vi "标准化行结束符.vi"(4 "End Of Line (Native)":T1(ring) caption="EOL(Native)", 7 "String In":string caption="字符串输入") -> (2 "String Out":string caption="字符串输出")   [LabVIEW 2012]
doc: "Converts the line endings of <B>String In</B> from whatever they are to the type indicated in <B>End Of Line</B>.\n\n<B>String In</B> - The string to convert.\n<B>String Out</B> - The string with the line endings changed.\n<B>End Of Line</B> - The type of line ending to convert to.\n\n<B>Native</B> is the native line ending (ie DOS \\r\\n, UNIX \\n, Mac \\r). <B>Native Command Line</B> is the appropriate of line ending when working with the command line."
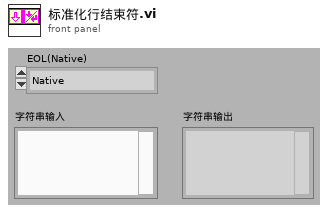
[diagram p1: front panel]
types:
  T1 = enum16{"Native", "Native Command Line", "UNIX", "Macintosh", "DOS"}
  T2 = enum32{"invalid OS target", "Mac OS", "Windows 3.1", "Windows 95/NT", "Solaris 1", "Solaris 2", "HP-UX", "PowerMAX", "Linux", "Irix", "Rhapsody", "BeOS", "AIX", "OSF1", "VxWorks", "PharLap", "Carbon"}
  T3 = enum32{"invalid OS target", "Mac OS", "Windows 3.1", "Windows 95/NT", "Solaris 1", "Solaris 2", "HP-UX", "PowerMAX", "Linux", "Irix", "Rhapsody", "BeOS", "AIX", "OSF1", "VxWorks", "PharLap", "Carbon", "RTX", "Windows x64", "Linux x64"}
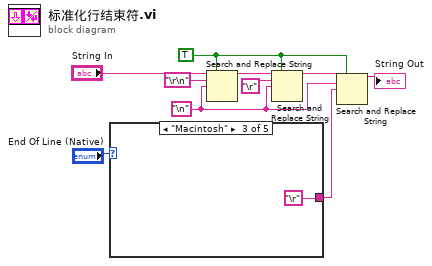
[diagram p0: block diagram]
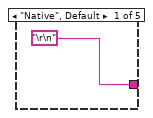
[diagram p2: hidden frame]
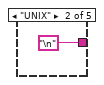
[diagram p3: hidden frame]
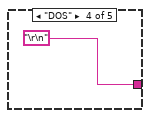
[diagram p4: hidden frame]
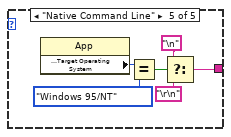
[diagram p5: hidden frame]
diagram:
  w3 = "\n" ("search string")
  w4 = TRUE ("replace all? (F)")
  n1 = case shown="\"Macintosh\"" "End Of Line (Native)" {
    tunnel: ["\r\n" "\n" "\r" "\r\n" w15] -> w2
    frame "Native", Default {
    }
    frame "UNIX" {
    }
    frame "Macintosh" {
    }
    frame "DOS" {
    }
    frame "Native Command Line" {
      n2 = property class="App"() -> ("Application:Target Operating System"=w20:T3)  [unwired: 2 in, 2 out]
      n3 = Equal?(x=w20, y=T2."Windows 95/NT" ("Application:Target Operating System")) -> (x = y?=w18:bool)
      n4 = Select(t="\n" ("search string"), s=w18, f="\r\n") -> (s? t:f=w15:string)
    }
  }
  n5 = Search and Replace String(replace all?=w4, input string="String In", search string="\r\n", replace string=w3) -> (result string=w8:string)  [unwired: 4 in, 3 out]
  n6 = Search and Replace String(replace all?=w4, input string=w8, search string="\r", replace string=w3) -> (result string=w5:string)  [unwired: 4 in, 3 out]
  n7 = Search and Replace String(replace all?=w4, input string=w5, search string=w3, replace string=w2) -> (result string=→"String Out":string)  [unwired: 4 in, 3 out]
